vi "input to tag bus.vi"(9 "indices":T1, 10 "data cluster":T2, 11 "tag bus in":T3) -> (3 "tag bus out":T3)   [LabVIEW 2017, in "GPIC Core runtime.lvclass"]
uses:
  GPIC Core runtime.lvclass
  <vilib>/NI/Tag Bus/table/data table.ctl
  input user data.ctl
  configuration/input data indices.ctl
  <vilib>/NI/Tag Bus/table/data polymorphs/write one/write Boolean.vi
  <vilib>/NI/Tag Bus/table/data polymorphs/write one/write Single.vi
  <vilib>/NI/Tag Bus/table/data polymorphs/write one/write I16.vi
  <vilib>/NI/Tag Bus/table/data table.lvlib
  configuration/GPIC Core configuration.lvclass
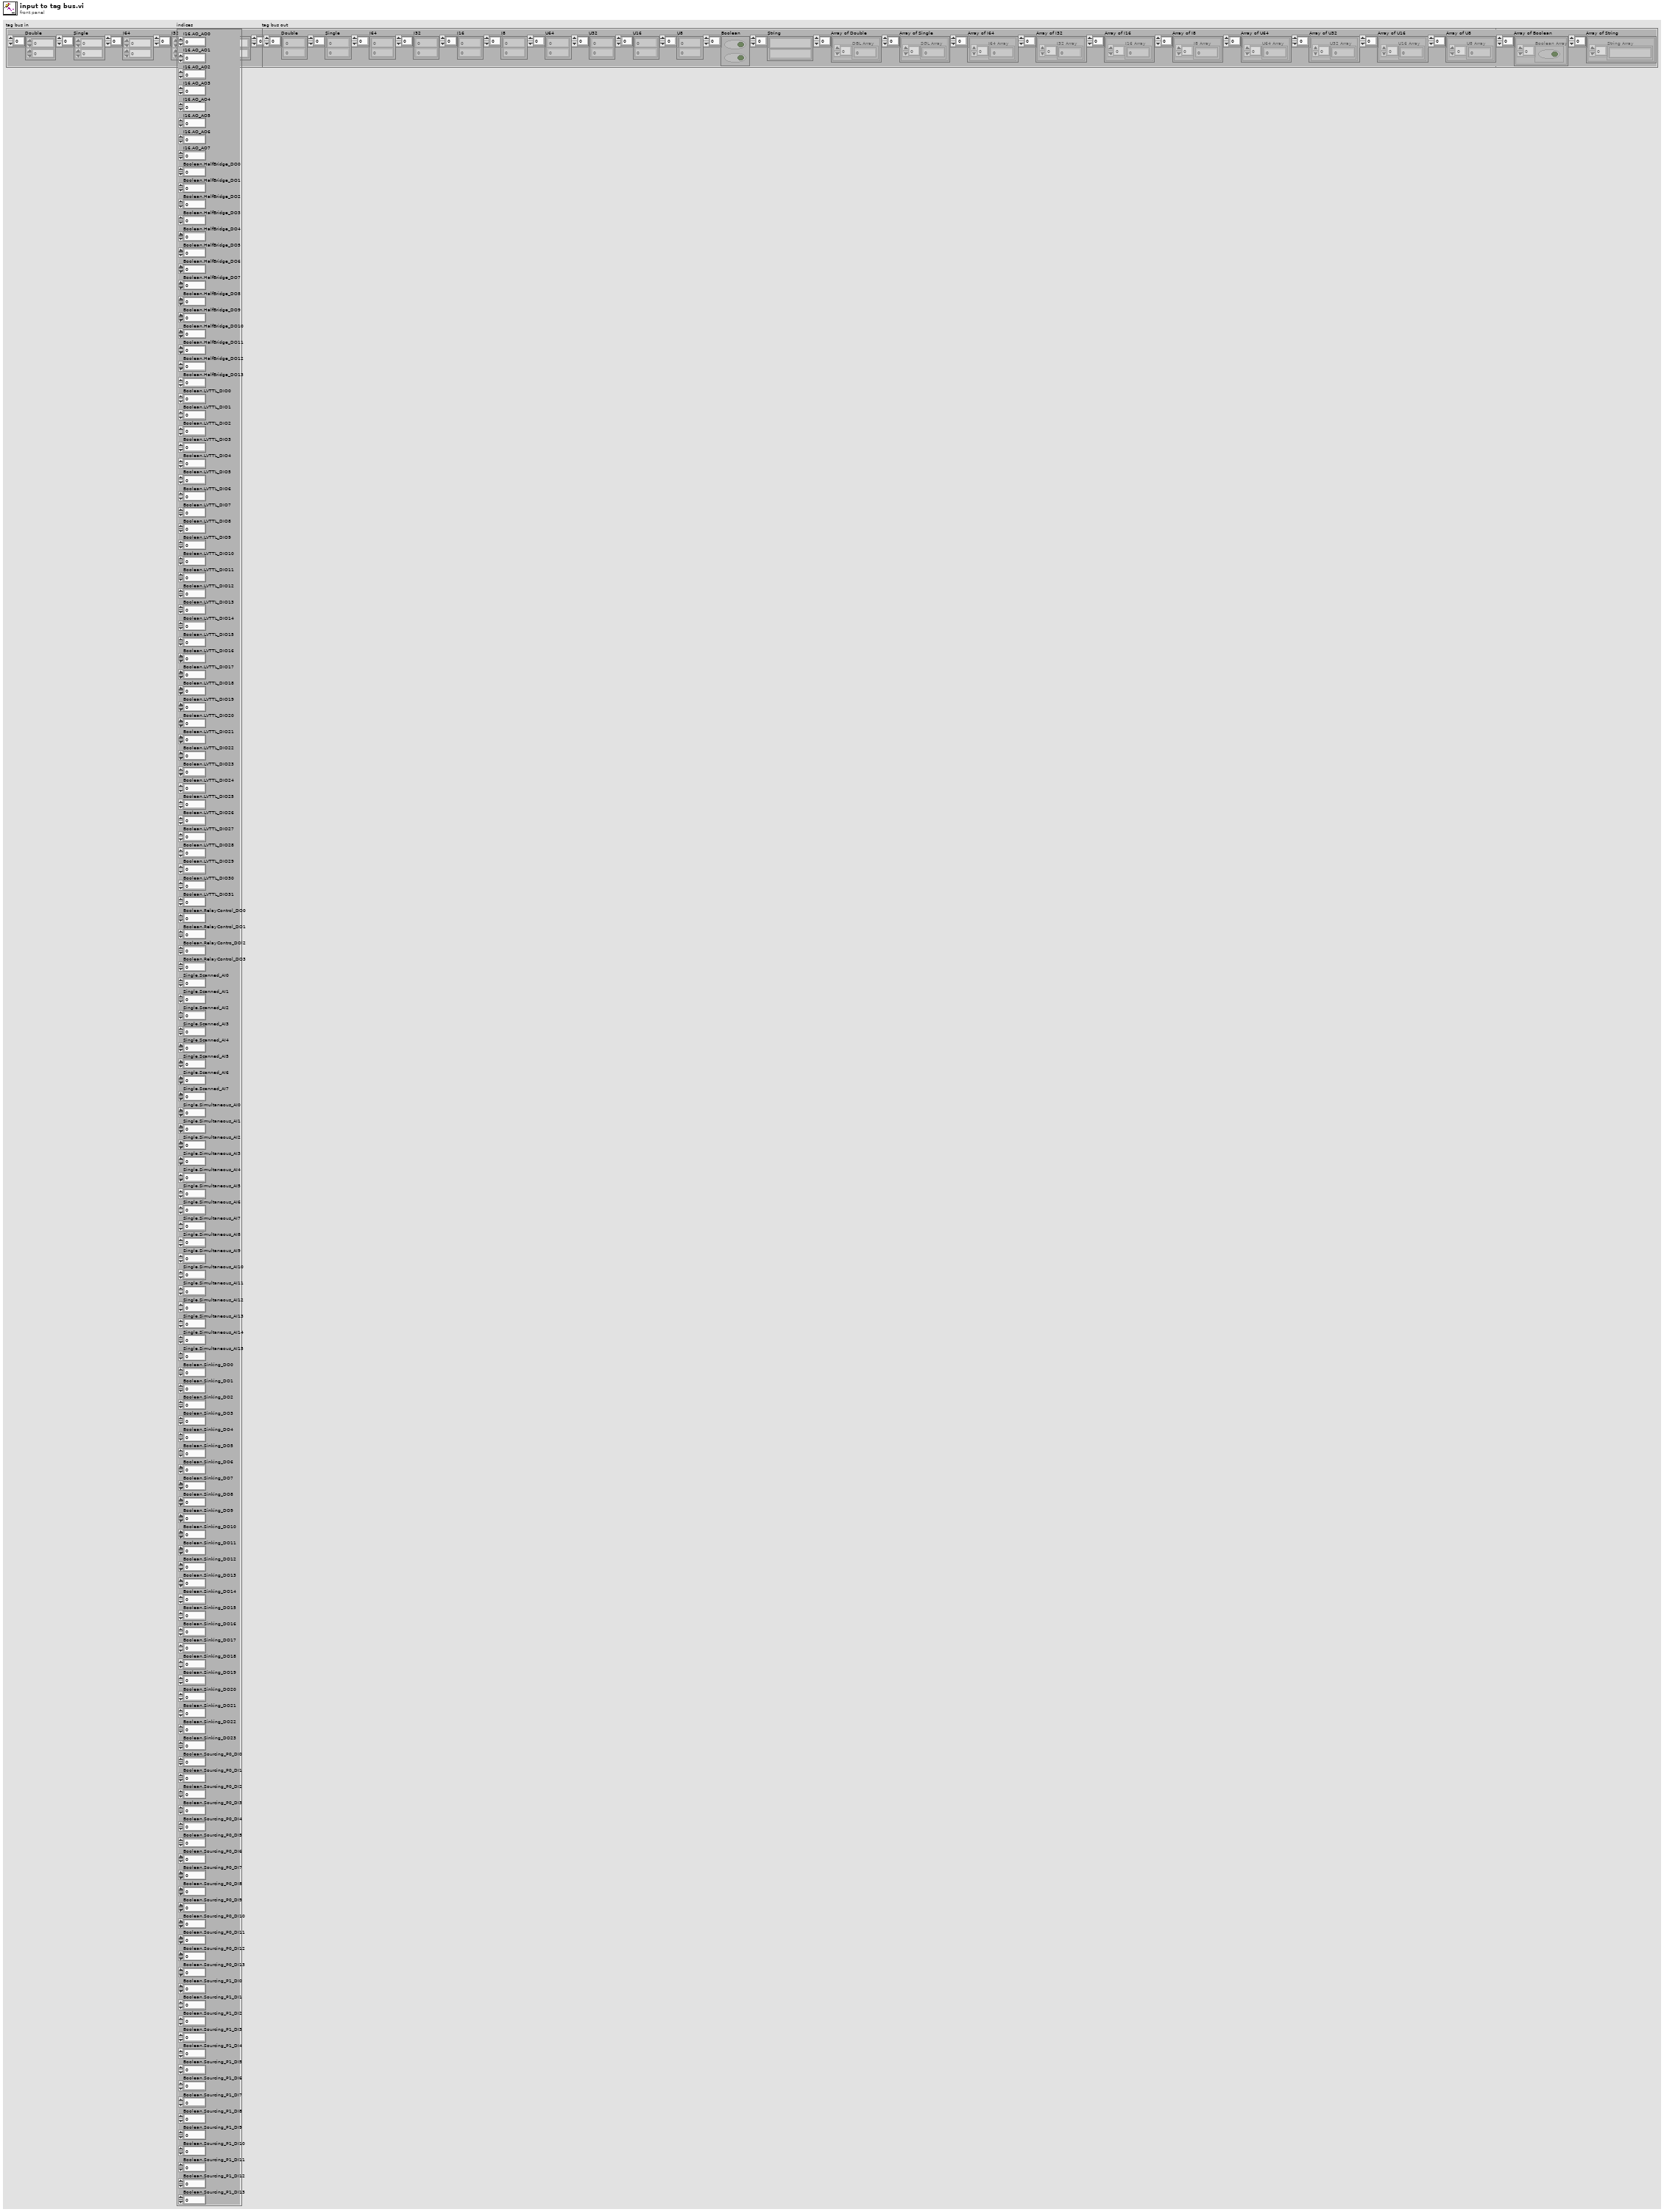
[diagram p1: front panel]
types:
  T1 = typedef "GPIC Core configuration.lvclass/input data indices.ctl" = cluster{"I16.AO_AO0":i32, "I16.AO_AO1":i32, "I16.AO_AO2":i32, "I16.AO_AO3":i32, "I16.AO_AO4":i32, "I16.AO_AO5":i32, "I16.AO_AO6":i32, "I16.AO_AO7":i32, "Boolean.HalfBridge_DO0":i32, "Boolean.HalfBridge_DO1":i32, "Boolean.HalfBridge_DO2":i32, "Boolean.HalfBridge_DO3":i32, "Boolean.HalfBridge_DO4":i32, "Boolean.HalfBridge_DO5":i32, "Boolean.HalfBridge_DO6":i32, "Boolean.HalfBridge_DO7":i32, "Boolean.HalfBridge_DO8":i32, "Boolean.HalfBridge_DO9":i32, "Boolean.HalfBridge_DO10":i32, "Boolean.HalfBridge_DO11":i32, "Boolean.HalfBridge_DO12":i32, "Boolean.HalfBridge_DO13":i32, "Boolean.LVTTL_DIO0":i32, "Boolean.LVTTL_DIO1":i32, "Boolean.LVTTL_DIO2":i32, "Boolean.LVTTL_DIO3":i32, "Boolean.LVTTL_DIO4":i32, "Boolean.LVTTL_DIO5":i32, "Boolean.LVTTL_DIO6":i32, "Boolean.LVTTL_DIO7":i32, "Boolean.LVTTL_DIO8":i32, "Boolean.LVTTL_DIO9":i32, "Boolean.LVTTL_DIO10":i32, "Boolean.LVTTL_DIO11":i32, "Boolean.LVTTL_DIO12":i32, "Boolean.LVTTL_DIO13":i32, "Boolean.LVTTL_DIO14":i32, "Boolean.LVTTL_DIO15":i32, "Boolean.LVTTL_DIO16":i32, "Boolean.LVTTL_DIO17":i32, "Boolean.LVTTL_DIO18":i32, "Boolean.LVTTL_DIO19":i32, "Boolean.LVTTL_DIO20":i32, "Boolean.LVTTL_DIO21":i32, "Boolean.LVTTL_DIO22":i32, "Boolean.LVTTL_DIO23":i32, "Boolean.LVTTL_DIO24":i32, "Boolean.LVTTL_DIO25":i32, "Boolean.LVTTL_DIO26":i32, "Boolean.LVTTL_DIO27":i32, "Boolean.LVTTL_DIO28":i32, "Boolean.LVTTL_DIO29":i32, "Boolean.LVTTL_DIO30":i32, "Boolean.LVTTL_DIO31":i32, "Boolean.RelayControl_DO0":i32, "Boolean.RelayControl_DO1":i32, "Boolean.RelayContro_DOl2":i32, "Boolean.RelayControl_DO3":i32, "Single.Scanned_AI0":i32, "Single.Scanned_AI1":i32, "Single.Scanned_AI2":i32, "Single.Scanned_AI3":i32, "Single.Scanned_AI4":i32, "Single.Scanned_AI5":i32, "Single.Scanned_AI6":i32, "Single.Scanned_AI7":i32, "Single.Simultaneous_AI0":i32, "Single.Simultaneous_AI1":i32, "Single.Simultaneous_AI2":i32, "Single.Simultaneous_AI3":i32, "Single.Simultaneous_AI4":i32, "Single.Simultaneous_AI5":i32, "Single.Simultaneous_AI6":i32, "Single.Simultaneous_AI7":i32, "Single.Simultaneous_AI8":i32, "Single.Simultaneous_AI9":i32, "Single.Simultaneous_AI10":i32, "Single.Simultaneous_AI11":i32, "Single.Simultaneous_AI12":i32, "Single.Simultaneous_AI13":i32, "Single.Simultaneous_AI14":i32, "Single.Simultaneous_AI15":i32, "Boolean.Sinking_DO0":i32, "Boolean.Sinking_DO1":i32, "Boolean.Sinking_DO2":i32, "Boolean.Sinking_DO3":i32, "Boolean.Sinking_DO4":i32, "Boolean.Sinking_DO5":i32, "Boolean.Sinking_DO6":i32, "Boolean.Sinking_DO7":i32, "Boolean.Sinking_DO8":i32, "Boolean.Sinking_DO9":i32, "Boolean.Sinking_DO10":i32, "Boolean.Sinking_DO11":i32, "Boolean.Sinking_DO12":i32, "Boolean.Sinking_DO13":i32, "Boolean.Sinking_DO14":i32, "Boolean.Sinking_DO15":i32, "Boolean.Sinking_DO16":i32, "Boolean.Sinking_DO17":i32, "Boolean.Sinking_DO18":i32, "Boolean.Sinking_DO19":i32, "Boolean.Sinking_DO20":i32, "Boolean.Sinking_DO21":i32, "Boolean.Sinking_DO22":i32, "Boolean.Sinking_DO23":i32, "Boolean.Sourcing_P0_DI0":i32, "Boolean.Sourcing_P0_DI1":i32, "Boolean.Sourcing_P0_DI2":i32, "Boolean.Sourcing_P0_DI3":i32, "Boolean.Sourcing_P0_DI4":i32, "Boolean.Sourcing_P0_DI5":i32, "Boolean.Sourcing_P0_DI6":i32, "Boolean.Sourcing_P0_DI7":i32, "Boolean.Sourcing_P0_DI8":i32, "Boolean.Sourcing_P0_DI9":i32, "Boolean.Sourcing_P0_DI10":i32, "Boolean.Sourcing_P0_DI11":i32, "Boolean.Sourcing_P0_DI12":i32, "Boolean.Sourcing_P0_DI13":i32, "Boolean.Sourcing_P1_DI0":i32, "Boolean.Sourcing_P1_DI1":i32, "Boolean.Sourcing_P1_DI2":i32, "Boolean.Sourcing_P1_DI3":i32, "Boolean.Sourcing_P1_DI4":i32, "Boolean.Sourcing_P1_DI5":i32, "Boolean.Sourcing_P1_DI6":i32, "Boolean.Sourcing_P1_DI7":i32, "Boolean.Sourcing_P1_DI8":i32, "Boolean.Sourcing_P1_DI9":i32, "Boolean.Sourcing_P1_DI10":i32, "Boolean.Sourcing_P1_DI11":i32, "Boolean.Sourcing_P1_DI12":i32, "Boolean.Sourcing_P1_DI13":i32}
  T2 = typedef "GPIC Core runtime.lvclass/input user data.ctl" = cluster{"AO_AO0":i16, "AO_AO1":i16, "AO_AO2":i16, "AO_AO3":i16, "AO_AO4":i16, "AO_AO5":i16, "AO_AO6":i16, "AO_AO7":i16, "HalfBridge_DO0":bool, "HalfBridge_DO1":bool, "HalfBridge_DO2":bool, "HalfBridge_DO3":bool, "HalfBridge_DO4":bool, "HalfBridge_DO5":bool, "HalfBridge_DO6":bool, "HalfBridge_DO7":bool, "HalfBridge_DO8":bool, "HalfBridge_DO9":bool, "HalfBridge_DO10":bool, "HalfBridge_DO11":bool, "HalfBridge_DO12":bool, "HalfBridge_DO13":bool, "LVTTL_DIO0":bool, "LVTTL_DIO1":bool, "LVTTL_DIO2":bool, "LVTTL_DIO3":bool, "LVTTL_DIO4":bool, "LVTTL_DIO5":bool, "LVTTL_DIO6":bool, "LVTTL_DIO7":bool, "LVTTL_DIO8":bool, "LVTTL_DIO9":bool, "LVTTL_DIO10":bool, "LVTTL_DIO11":bool, "LVTTL_DIO12":bool, "LVTTL_DIO13":bool, "LVTTL_DIO14":bool, "LVTTL_DIO15":bool, "LVTTL_DIO16":bool, "LVTTL_DIO17":bool, "LVTTL_DIO18":bool, "LVTTL_DIO19":bool, "LVTTL_DIO20":bool, "LVTTL_DIO21":bool, "LVTTL_DIO22":bool, "LVTTL_DIO23":bool, "LVTTL_DIO24":bool, "LVTTL_DIO25":bool, "LVTTL_DIO26":bool, "LVTTL_DIO27":bool, "LVTTL_DIO28":bool, "LVTTL_DIO29":bool, "LVTTL_DIO30":bool, "LVTTL_DIO31":bool, "RelayControl_DO0":bool, "RelayControl_DO1":bool, "RelayContro_DOl2":bool, "RelayControl_DO3":bool, "Scanned_AI0":sgl, "Scanned_AI1":sgl, "Scanned_AI2":sgl, "Scanned_AI3":sgl, "Scanned_AI4":sgl, "Scanned_AI5":sgl, "Scanned_AI6":sgl, "Scanned_AI7":sgl, "Simultaneous_AI0":sgl, "Simultaneous_AI1":sgl, "Simultaneous_AI2":sgl, "Simultaneous_AI3":sgl, "Simultaneous_AI4":sgl, "Simultaneous_AI5":sgl, "Simultaneous_AI6":sgl, "Simultaneous_AI7":sgl, "Simultaneous_AI8":sgl, "Simultaneous_AI9":sgl, "Simultaneous_AI10":sgl, "Simultaneous_AI11":sgl, "Simultaneous_AI12":sgl, "Simultaneous_AI13":sgl, "Simultaneous_AI14":sgl, "Simultaneous_AI15":sgl, "Sinking_DO0":bool, "Sinking_DO1":bool, "Sinking_DO2":bool, "Sinking_DO3":bool, "Sinking_DO4":bool, "Sinking_DO5":bool, "Sinking_DO6":bool, "Sinking_DO7":bool, "Sinking_DO8":bool, "Sinking_DO9":bool, "Sinking_DO10":bool, "Sinking_DO11":bool, "Sinking_DO12":bool, "Sinking_DO13":bool, "Sinking_DO14":bool, "Sinking_DO15":bool, "Sinking_DO16":bool, "Sinking_DO17":bool, "Sinking_DO18":bool, "Sinking_DO19":bool, "Sinking_DO20":bool, "Sinking_DO21":bool, "Sinking_DO22":bool, "Sinking_DO23":bool, "Sourcing_P0_DI0":bool, "Sourcing_P0_DI1":bool, "Sourcing_P0_DI2":bool, "Sourcing_P0_DI3":bool, "Sourcing_P0_DI4":bool, "Sourcing_P0_DI5":bool, "Sourcing_P0_DI6":bool, "Sourcing_P0_DI7":bool, "Sourcing_P0_DI8":bool, "Sourcing_P0_DI9":bool, "Sourcing_P0_DI10":bool, "Sourcing_P0_DI11":bool, "Sourcing_P0_DI12":bool, "Sourcing_P0_DI13":bool, "Sourcing_P1_DI0":bool, "Sourcing_P1_DI1":bool, "Sourcing_P1_DI2":bool, "Sourcing_P1_DI3":bool, "Sourcing_P1_DI4":bool, "Sourcing_P1_DI5":bool, "Sourcing_P1_DI6":bool, "Sourcing_P1_DI7":bool, "Sourcing_P1_DI8":bool, "Sourcing_P1_DI9":bool, "Sourcing_P1_DI10":bool, "Sourcing_P1_DI11":bool, "Sourcing_P1_DI12":bool, "Sourcing_P1_DI13":bool}
  T3 = typedef "tag bus.lvlib/data table.lvlib/data table.ctl" = cluster{"Double":dbl[], "Single":sgl[], "I64":i64[], "I32":i32[], "I16":i16[], "I8":i8[], "U64":u64[], "U32":u32[], "U16":u16[], "U8":u8[], "Boolean":bool[], "String":string[], "Array of Double":cluster{"DBL Array":dbl[]}[], "Array of Single":cluster{"SGL Array":sgl[]}[], "Array of I64":cluster{"I64 Array":i64[]}[], "Array of I32":cluster{"I32 Array":i32[]}[], "Array of I16":cluster{"I16 Array":i16[]}[], "Array of I8":cluster{"I8 Array":i8[]}[], "Array of U64":cluster{"U64 Array":u64[]}[], "Array of U32":cluster{"U32 Array":u32[]}[], "Array of U16":cluster{"U16 Array":u16[]}[], "Array of U8":cluster{"U8 Array":u8[]}[], "Array of Boolean":cluster{"Boolean Array":bool[]}[], "Array of String":cluster{"String Array":string[]}[]}
diagram:
  n1 = Unbundle By Name("indices") -> ("I16.AO_AO0"=w4:i32, "I16.AO_AO1"=w7:i32, "I16.AO_AO2"=w10:i32, "I16.AO_AO3"=w13:i32, "I16.AO_AO4"=w16:i32, "I16.AO_AO5"=w19:i32, "I16.AO_AO6"=w22:i32, "I16.AO_AO7"=w25:i32, "Boolean.HalfBridge_DO0"=w28:i32, "Boolean.HalfBridge_DO1"=w31:i32, "Boolean.HalfBridge_DO2"=w34:i32, "Boolean.HalfBridge_DO3"=w37:i32, "Boolean.HalfBridge_DO4"=w40:i32, "Boolean.HalfBridge_DO5"=w43:i32, "Boolean.HalfBridge_DO6"=w46:i32, "Boolean.HalfBridge_DO7"=w49:i32, "Boolean.HalfBridge_DO8"=w52:i32, "Boolean.HalfBridge_DO9"=w55:i32, "Boolean.HalfBridge_DO10"=w58:i32, "Boolean.HalfBridge_DO11"=w61:i32, "Boolean.HalfBridge_DO12"=w64:i32, "Boolean.HalfBridge_DO13"=w67:i32, "Boolean.LVTTL_DIO0"=w70:i32, "Boolean.LVTTL_DIO1"=w73:i32, "Boolean.LVTTL_DIO2"=w76:i32, "Boolean.LVTTL_DIO3"=w79:i32, "Boolean.LVTTL_DIO4"=w82:i32, "Boolean.LVTTL_DIO5"=w85:i32, "Boolean.LVTTL_DIO6"=w88:i32, "Boolean.LVTTL_DIO7"=w91:i32, "Boolean.LVTTL_DIO8"=w94:i32, "Boolean.LVTTL_DIO9"=w97:i32, "Boolean.LVTTL_DIO10"=w100:i32, "Boolean.LVTTL_DIO11"=w103:i32, "Boolean.LVTTL_DIO12"=w106:i32, "Boolean.LVTTL_DIO13"=w109:i32, "Boolean.LVTTL_DIO14"=w112:i32, "Boolean.LVTTL_DIO15"=w115:i32, "Boolean.LVTTL_DIO16"=w118:i32, "Boolean.LVTTL_DIO17"=w121:i32, "Boolean.LVTTL_DIO18"=w124:i32, "Boolean.LVTTL_DIO19"=w127:i32, "Boolean.LVTTL_DIO20"=w130:i32, "Boolean.LVTTL_DIO21"=w133:i32, "Boolean.LVTTL_DIO22"=w136:i32, "Boolean.LVTTL_DIO23"=w139:i32, "Boolean.LVTTL_DIO24"=w142:i32, "Boolean.LVTTL_DIO25"=w145:i32, "Boolean.LVTTL_DIO26"=w148:i32, "Boolean.LVTTL_DIO27"=w151:i32, "Boolean.LVTTL_DIO28"=w154:i32, "Boolean.LVTTL_DIO29"=w157:i32, "Boolean.LVTTL_DIO30"=w160:i32, "Boolean.LVTTL_DIO31"=w163:i32, "Boolean.RelayControl_DO0"=w166:i32, "Boolean.RelayControl_DO1"=w169:i32, "Boolean.RelayContro_DOl2"=w172:i32, "Boolean.RelayControl_DO3"=w175:i32, "Single.Scanned_AI0"=w178:i32, "Single.Scanned_AI1"=w181:i32, "Single.Scanned_AI2"=w184:i32, "Single.Scanned_AI3"=w187:i32, "Single.Scanned_AI4"=w190:i32, "Single.Scanned_AI5"=w193:i32, "Single.Scanned_AI6"=w196:i32, "Single.Scanned_AI7"=w199:i32, "Single.Simultaneous_AI0"=w202:i32, "Single.Simultaneous_AI1"=w205:i32, "Single.Simultaneous_AI2"=w208:i32, "Single.Simultaneous_AI3"=w211:i32, "Single.Simultaneous_AI4"=w214:i32, "Single.Simultaneous_AI5"=w217:i32, "Single.Simultaneous_AI6"=w220:i32, "Single.Simultaneous_AI7"=w223:i32, "Single.Simultaneous_AI8"=w226:i32, "Single.Simultaneous_AI9"=w229:i32, "Single.Simultaneous_AI10"=w232:i32, "Single.Simultaneous_AI11"=w235:i32, "Single.Simultaneous_AI12"=w238:i32, "Single.Simultaneous_AI13"=w241:i32, "Single.Simultaneous_AI14"=w244:i32, "Single.Simultaneous_AI15"=w247:i32, "Boolean.Sinking_DO0"=w250:i32, "Boolean.Sinking_DO1"=w253:i32, "Boolean.Sinking_DO2"=w256:i32, "Boolean.Sinking_DO3"=w259:i32, "Boolean.Sinking_DO4"=w262:i32, "Boolean.Sinking_DO5"=w265:i32, "Boolean.Sinking_DO6"=w268:i32, "Boolean.Sinking_DO7"=w271:i32, "Boolean.Sinking_DO8"=w274:i32, "Boolean.Sinking_DO9"=w277:i32, "Boolean.Sinking_DO10"=w280:i32, "Boolean.Sinking_DO11"=w283:i32, "Boolean.Sinking_DO12"=w286:i32, "Boolean.Sinking_DO13"=w289:i32, "Boolean.Sinking_DO14"=w292:i32, "Boolean.Sinking_DO15"=w295:i32, "Boolean.Sinking_DO16"=w298:i32, "Boolean.Sinking_DO17"=w301:i32, "Boolean.Sinking_DO18"=w304:i32, "Boolean.Sinking_DO19"=w307:i32, "Boolean.Sinking_DO20"=w310:i32, "Boolean.Sinking_DO21"=w313:i32, "Boolean.Sinking_DO22"=w316:i32, "Boolean.Sinking_DO23"=w319:i32, "Boolean.Sourcing_P0_DI0"=w322:i32, "Boolean.Sourcing_P0_DI1"=w325:i32, "Boolean.Sourcing_P0_DI2"=w328:i32, "Boolean.Sourcing_P0_DI3"=w331:i32, "Boolean.Sourcing_P0_DI4"=w334:i32, "Boolean.Sourcing_P0_DI5"=w337:i32, "Boolean.Sourcing_P0_DI6"=w340:i32, "Boolean.Sourcing_P0_DI7"=w343:i32, "Boolean.Sourcing_P0_DI8"=w346:i32, "Boolean.Sourcing_P0_DI9"=w349:i32, "Boolean.Sourcing_P0_DI10"=w352:i32, "Boolean.Sourcing_P0_DI11"=w355:i32, "Boolean.Sourcing_P0_DI12"=w358:i32, "Boolean.Sourcing_P0_DI13"=w361:i32, "Boolean.Sourcing_P1_DI0"=w364:i32, "Boolean.Sourcing_P1_DI1"=w367:i32, "Boolean.Sourcing_P1_DI2"=w370:i32, "Boolean.Sourcing_P1_DI3"=w373:i32, "Boolean.Sourcing_P1_DI4"=w376:i32, "Boolean.Sourcing_P1_DI5"=w379:i32, "Boolean.Sourcing_P1_DI6"=w382:i32, "Boolean.Sourcing_P1_DI7"=w385:i32, "Boolean.Sourcing_P1_DI8"=w388:i32, "Boolean.Sourcing_P1_DI9"=w391:i32, "Boolean.Sourcing_P1_DI10"=w394:i32, "Boolean.Sourcing_P1_DI11"=w397:i32, "Boolean.Sourcing_P1_DI12"=w400:i32, "Boolean.Sourcing_P1_DI13"=w403:i32)
  n2 = Unbundle By Name("data cluster") -> ("AO_AO0"=w3:i16, "AO_AO1"=w6:i16, "AO_AO2"=w9:i16, "AO_AO3"=w12:i16, "AO_AO4"=w15:i16, "AO_AO5"=w18:i16, "AO_AO6"=w21:i16, "AO_AO7"=w24:i16, "HalfBridge_DO0"=w27:bool, "HalfBridge_DO1"=w30:bool, "HalfBridge_DO2"=w33:bool, "HalfBridge_DO3"=w36:bool, "HalfBridge_DO4"=w39:bool, "HalfBridge_DO5"=w42:bool, "HalfBridge_DO6"=w45:bool, "HalfBridge_DO7"=w48:bool, "HalfBridge_DO8"=w51:bool, "HalfBridge_DO9"=w54:bool, "HalfBridge_DO10"=w57:bool, "HalfBridge_DO11"=w60:bool, "HalfBridge_DO12"=w63:bool, "HalfBridge_DO13"=w66:bool, "LVTTL_DIO0"=w69:bool, "LVTTL_DIO1"=w72:bool, "LVTTL_DIO2"=w75:bool, "LVTTL_DIO3"=w78:bool, "LVTTL_DIO4"=w81:bool, "LVTTL_DIO5"=w84:bool, "LVTTL_DIO6"=w87:bool, "LVTTL_DIO7"=w90:bool, "LVTTL_DIO8"=w93:bool, "LVTTL_DIO9"=w96:bool, "LVTTL_DIO10"=w99:bool, "LVTTL_DIO11"=w102:bool, "LVTTL_DIO12"=w105:bool, "LVTTL_DIO13"=w108:bool, "LVTTL_DIO14"=w111:bool, "LVTTL_DIO15"=w114:bool, "LVTTL_DIO16"=w117:bool, "LVTTL_DIO17"=w120:bool, "LVTTL_DIO18"=w123:bool, "LVTTL_DIO19"=w126:bool, "LVTTL_DIO20"=w129:bool, "LVTTL_DIO21"=w132:bool, "LVTTL_DIO22"=w135:bool, "LVTTL_DIO23"=w138:bool, "LVTTL_DIO24"=w141:bool, "LVTTL_DIO25"=w144:bool, "LVTTL_DIO26"=w147:bool, "LVTTL_DIO27"=w150:bool, "LVTTL_DIO28"=w153:bool, "LVTTL_DIO29"=w156:bool, "LVTTL_DIO30"=w159:bool, "LVTTL_DIO31"=w162:bool, "RelayControl_DO0"=w165:bool, "RelayControl_DO1"=w168:bool, "RelayContro_DOl2"=w171:bool, "RelayControl_DO3"=w174:bool, "Scanned_AI0"=w177:sgl, "Scanned_AI1"=w180:sgl, "Scanned_AI2"=w183:sgl, "Scanned_AI3"=w186:sgl, "Scanned_AI4"=w189:sgl, "Scanned_AI5"=w192:sgl, "Scanned_AI6"=w195:sgl, "Scanned_AI7"=w198:sgl, "Simultaneous_AI0"=w201:sgl, "Simultaneous_AI1"=w204:sgl, "Simultaneous_AI2"=w207:sgl, "Simultaneous_AI3"=w210:sgl, "Simultaneous_AI4"=w213:sgl, "Simultaneous_AI5"=w216:sgl, "Simultaneous_AI6"=w219:sgl, "Simultaneous_AI7"=w222:sgl, "Simultaneous_AI8"=w225:sgl, "Simultaneous_AI9"=w228:sgl, "Simultaneous_AI10"=w231:sgl, "Simultaneous_AI11"=w234:sgl, "Simultaneous_AI12"=w237:sgl, "Simultaneous_AI13"=w240:sgl, "Simultaneous_AI14"=w243:sgl, "Simultaneous_AI15"=w246:sgl, "Sinking_DO0"=w249:bool, "Sinking_DO1"=w252:bool, "Sinking_DO2"=w255:bool, "Sinking_DO3"=w258:bool, "Sinking_DO4"=w261:bool, "Sinking_DO5"=w264:bool, "Sinking_DO6"=w267:bool, "Sinking_DO7"=w270:bool, "Sinking_DO8"=w273:bool, "Sinking_DO9"=w276:bool, "Sinking_DO10"=w279:bool, "Sinking_DO11"=w282:bool, "Sinking_DO12"=w285:bool, "Sinking_DO13"=w288:bool, "Sinking_DO14"=w291:bool, "Sinking_DO15"=w294:bool, "Sinking_DO16"=w297:bool, "Sinking_DO17"=w300:bool, "Sinking_DO18"=w303:bool, "Sinking_DO19"=w306:bool, "Sinking_DO20"=w309:bool, "Sinking_DO21"=w312:bool, "Sinking_DO22"=w315:bool, "Sinking_DO23"=w318:bool, "Sourcing_P0_DI0"=w321:bool, "Sourcing_P0_DI1"=w324:bool, "Sourcing_P0_DI2"=w327:bool, "Sourcing_P0_DI3"=w330:bool, "Sourcing_P0_DI4"=w333:bool, "Sourcing_P0_DI5"=w336:bool, "Sourcing_P0_DI6"=w339:bool, "Sourcing_P0_DI7"=w342:bool, "Sourcing_P0_DI8"=w345:bool, "Sourcing_P0_DI9"=w348:bool, "Sourcing_P0_DI10"=w351:bool, "Sourcing_P0_DI11"=w354:bool, "Sourcing_P0_DI12"=w357:bool, "Sourcing_P0_DI13"=w360:bool, "Sourcing_P1_DI0"=w363:bool, "Sourcing_P1_DI1"=w366:bool, "Sourcing_P1_DI2"=w369:bool, "Sourcing_P1_DI3"=w372:bool, "Sourcing_P1_DI4"=w375:bool, "Sourcing_P1_DI5"=w378:bool, "Sourcing_P1_DI6"=w381:bool, "Sourcing_P1_DI7"=w384:bool, "Sourcing_P1_DI8"=w387:bool, "Sourcing_P1_DI9"=w390:bool, "Sourcing_P1_DI10"=w393:bool, "Sourcing_P1_DI11"=w396:bool, "Sourcing_P1_DI12"=w399:bool, "Sourcing_P1_DI13"=w402:bool)
  n3 = call-poly <vilib>:"write data element.vi"("value"=w402, "index"=w403, "data table in"="tag bus in") -> ("data table out"=w398:T3)  [unwired: 8 in]
  n4 = call-poly <vilib>:"write data element.vi"("value"=w399, "index"=w400, "data table in"=w398) -> ("data table out"=w395:T3)  [unwired: 8 in]
  n5 = call-poly <vilib>:"write data element.vi"("value"=w396, "index"=w397, "data table in"=w395) -> ("data table out"=w392:T3)  [unwired: 8 in]
  n6 = call-poly <vilib>:"write data element.vi"("value"=w393, "index"=w394, "data table in"=w392) -> ("data table out"=w389:T3)  [unwired: 8 in]
  n7 = call-poly <vilib>:"write data element.vi"("value"=w390, "index"=w391, "data table in"=w389) -> ("data table out"=w386:T3)  [unwired: 8 in]
  n8 = call-poly <vilib>:"write data element.vi"("value"=w387, "index"=w388, "data table in"=w386) -> ("data table out"=w383:T3)  [unwired: 8 in]
  n9 = call-poly <vilib>:"write data element.vi"("value"=w384, "index"=w385, "data table in"=w383) -> ("data table out"=w380:T3)  [unwired: 8 in]
  n10 = call-poly <vilib>:"write data element.vi"("value"=w381, "index"=w382, "data table in"=w380) -> ("data table out"=w377:T3)  [unwired: 8 in]
  n11 = call-poly <vilib>:"write data element.vi"("value"=w378, "index"=w379, "data table in"=w377) -> ("data table out"=w374:T3)  [unwired: 8 in]
  n12 = call-poly <vilib>:"write data element.vi"("value"=w375, "index"=w376, "data table in"=w374) -> ("data table out"=w371:T3)  [unwired: 8 in]
  n13 = call-poly <vilib>:"write data element.vi"("value"=w372, "index"=w373, "data table in"=w371) -> ("data table out"=w368:T3)  [unwired: 8 in]
  n14 = call-poly <vilib>:"write data element.vi"("value"=w369, "index"=w370, "data table in"=w368) -> ("data table out"=w365:T3)  [unwired: 8 in]
  n15 = call-poly <vilib>:"write data element.vi"("value"=w366, "index"=w367, "data table in"=w365) -> ("data table out"=w362:T3)  [unwired: 8 in]
  n16 = call-poly <vilib>:"write data element.vi"("value"=w363, "index"=w364, "data table in"=w362) -> ("data table out"=w359:T3)  [unwired: 8 in]
  n17 = call-poly <vilib>:"write data element.vi"("value"=w360, "index"=w361, "data table in"=w359) -> ("data table out"=w356:T3)  [unwired: 8 in]
  n18 = call-poly <vilib>:"write data element.vi"("value"=w357, "index"=w358, "data table in"=w356) -> ("data table out"=w353:T3)  [unwired: 8 in]
  n19 = call-poly <vilib>:"write data element.vi"("value"=w354, "index"=w355, "data table in"=w353) -> ("data table out"=w350:T3)  [unwired: 8 in]
  n20 = call-poly <vilib>:"write data element.vi"("value"=w351, "index"=w352, "data table in"=w350) -> ("data table out"=w347:T3)  [unwired: 8 in]
  n21 = call-poly <vilib>:"write data element.vi"("value"=w348, "index"=w349, "data table in"=w347) -> ("data table out"=w344:T3)  [unwired: 8 in]
  n22 = call-poly <vilib>:"write data element.vi"("value"=w345, "index"=w346, "data table in"=w344) -> ("data table out"=w341:T3)  [unwired: 8 in]
  n23 = call-poly <vilib>:"write data element.vi"("value"=w342, "index"=w343, "data table in"=w341) -> ("data table out"=w338:T3)  [unwired: 8 in]
  n24 = call-poly <vilib>:"write data element.vi"("value"=w339, "index"=w340, "data table in"=w338) -> ("data table out"=w335:T3)  [unwired: 8 in]
  n25 = call-poly <vilib>:"write data element.vi"("value"=w336, "index"=w337, "data table in"=w335) -> ("data table out"=w332:T3)  [unwired: 8 in]
  n26 = call-poly <vilib>:"write data element.vi"("value"=w333, "index"=w334, "data table in"=w332) -> ("data table out"=w329:T3)  [unwired: 8 in]
  n27 = call-poly <vilib>:"write data element.vi"("value"=w330, "index"=w331, "data table in"=w329) -> ("data table out"=w326:T3)  [unwired: 8 in]
  n28 = call-poly <vilib>:"write data element.vi"("value"=w327, "index"=w328, "data table in"=w326) -> ("data table out"=w323:T3)  [unwired: 8 in]
  n29 = call-poly <vilib>:"write data element.vi"("value"=w324, "index"=w325, "data table in"=w323) -> ("data table out"=w320:T3)  [unwired: 8 in]
  n30 = call-poly <vilib>:"write data element.vi"("value"=w321, "index"=w322, "data table in"=w320) -> ("data table out"=w317:T3)  [unwired: 8 in]
  n31 = call-poly <vilib>:"write data element.vi"("value"=w318, "index"=w319, "data table in"=w317) -> ("data table out"=w314:T3)  [unwired: 8 in]
  n32 = call-poly <vilib>:"write data element.vi"("value"=w315, "index"=w316, "data table in"=w314) -> ("data table out"=w311:T3)  [unwired: 8 in]
  n33 = call-poly <vilib>:"write data element.vi"("value"=w312, "index"=w313, "data table in"=w311) -> ("data table out"=w308:T3)  [unwired: 8 in]
  n34 = call-poly <vilib>:"write data element.vi"("value"=w309, "index"=w310, "data table in"=w308) -> ("data table out"=w305:T3)  [unwired: 8 in]
  n35 = call-poly <vilib>:"write data element.vi"("value"=w306, "index"=w307, "data table in"=w305) -> ("data table out"=w302:T3)  [unwired: 8 in]
  n36 = call-poly <vilib>:"write data element.vi"("value"=w303, "index"=w304, "data table in"=w302) -> ("data table out"=w299:T3)  [unwired: 8 in]
  n37 = call-poly <vilib>:"write data element.vi"("value"=w300, "index"=w301, "data table in"=w299) -> ("data table out"=w296:T3)  [unwired: 8 in]
  n38 = call-poly <vilib>:"write data element.vi"("value"=w297, "index"=w298, "data table in"=w296) -> ("data table out"=w293:T3)  [unwired: 8 in]
  n39 = call-poly <vilib>:"write data element.vi"("value"=w294, "index"=w295, "data table in"=w293) -> ("data table out"=w290:T3)  [unwired: 8 in]
  n40 = call-poly <vilib>:"write data element.vi"("value"=w291, "index"=w292, "data table in"=w290) -> ("data table out"=w287:T3)  [unwired: 8 in]
  n41 = call-poly <vilib>:"write data element.vi"("value"=w288, "index"=w289, "data table in"=w287) -> ("data table out"=w284:T3)  [unwired: 8 in]
  n42 = call-poly <vilib>:"write data element.vi"("value"=w285, "index"=w286, "data table in"=w284) -> ("data table out"=w281:T3)  [unwired: 8 in]
  n43 = call-poly <vilib>:"write data element.vi"("value"=w282, "index"=w283, "data table in"=w281) -> ("data table out"=w278:T3)  [unwired: 8 in]
  n44 = call-poly <vilib>:"write data element.vi"("value"=w279, "index"=w280, "data table in"=w278) -> ("data table out"=w275:T3)  [unwired: 8 in]
  n45 = call-poly <vilib>:"write data element.vi"("value"=w276, "index"=w277, "data table in"=w275) -> ("data table out"=w272:T3)  [unwired: 8 in]
  n46 = call-poly <vilib>:"write data element.vi"("value"=w273, "index"=w274, "data table in"=w272) -> ("data table out"=w269:T3)  [unwired: 8 in]
  n47 = call-poly <vilib>:"write data element.vi"("value"=w270, "index"=w271, "data table in"=w269) -> ("data table out"=w266:T3)  [unwired: 8 in]
  n48 = call-poly <vilib>:"write data element.vi"("value"=w267, "index"=w268, "data table in"=w266) -> ("data table out"=w263:T3)  [unwired: 8 in]
  n49 = call-poly <vilib>:"write data element.vi"("value"=w264, "index"=w265, "data table in"=w263) -> ("data table out"=w260:T3)  [unwired: 8 in]
  n50 = call-poly <vilib>:"write data element.vi"("value"=w261, "index"=w262, "data table in"=w260) -> ("data table out"=w257:T3)  [unwired: 8 in]
  n51 = call-poly <vilib>:"write data element.vi"("value"=w258, "index"=w259, "data table in"=w257) -> ("data table out"=w254:T3)  [unwired: 8 in]
  n52 = call-poly <vilib>:"write data element.vi"("value"=w255, "index"=w256, "data table in"=w254) -> ("data table out"=w251:T3)  [unwired: 8 in]
  n53 = call-poly <vilib>:"write data element.vi"("value"=w252, "index"=w253, "data table in"=w251) -> ("data table out"=w248:T3)  [unwired: 8 in]
  n54 = call-poly <vilib>:"write data element.vi"("value"=w249, "index"=w250, "data table in"=w248) -> ("data table out"=w245:T3)  [unwired: 8 in]
  n55 = call-poly <vilib>:"write data element.vi"("value"=w246, "index"=w247, "data table in"=w245) -> ("data table out"=w242:T3)  [unwired: 8 in]
  n56 = call-poly <vilib>:"write data element.vi"("value"=w243, "index"=w244, "data table in"=w242) -> ("data table out"=w239:T3)  [unwired: 8 in]
  n57 = call-poly <vilib>:"write data element.vi"("value"=w240, "index"=w241, "data table in"=w239) -> ("data table out"=w236:T3)  [unwired: 8 in]
  n58 = call-poly <vilib>:"write data element.vi"("value"=w237, "index"=w238, "data table in"=w236) -> ("data table out"=w233:T3)  [unwired: 8 in]
  n59 = call-poly <vilib>:"write data element.vi"("value"=w234, "index"=w235, "data table in"=w233) -> ("data table out"=w230:T3)  [unwired: 8 in]
  n60 = call-poly <vilib>:"write data element.vi"("value"=w231, "index"=w232, "data table in"=w230) -> ("data table out"=w227:T3)  [unwired: 8 in]
  n61 = call-poly <vilib>:"write data element.vi"("value"=w228, "index"=w229, "data table in"=w227) -> ("data table out"=w224:T3)  [unwired: 8 in]
  n62 = call-poly <vilib>:"write data element.vi"("value"=w225, "index"=w226, "data table in"=w224) -> ("data table out"=w221:T3)  [unwired: 8 in]
  n63 = call-poly <vilib>:"write data element.vi"("value"=w222, "index"=w223, "data table in"=w221) -> ("data table out"=w218:T3)  [unwired: 8 in]
  n64 = call-poly <vilib>:"write data element.vi"("value"=w219, "index"=w220, "data table in"=w218) -> ("data table out"=w215:T3)  [unwired: 8 in]
  n65 = call-poly <vilib>:"write data element.vi"("value"=w216, "index"=w217, "data table in"=w215) -> ("data table out"=w212:T3)  [unwired: 8 in]
  n66 = call-poly <vilib>:"write data element.vi"("value"=w213, "index"=w214, "data table in"=w212) -> ("data table out"=w209:T3)  [unwired: 8 in]
  n67 = call-poly <vilib>:"write data element.vi"("value"=w210, "index"=w211, "data table in"=w209) -> ("data table out"=w206:T3)  [unwired: 8 in]
  n68 = call-poly <vilib>:"write data element.vi"("value"=w207, "index"=w208, "data table in"=w206) -> ("data table out"=w203:T3)  [unwired: 8 in]
  n69 = call-poly <vilib>:"write data element.vi"("value"=w204, "index"=w205, "data table in"=w203) -> ("data table out"=w200:T3)  [unwired: 8 in]
  n70 = call-poly <vilib>:"write data element.vi"("value"=w201, "index"=w202, "data table in"=w200) -> ("data table out"=w197:T3)  [unwired: 8 in]
  n71 = call-poly <vilib>:"write data element.vi"("value"=w198, "index"=w199, "data table in"=w197) -> ("data table out"=w194:T3)  [unwired: 8 in]
  n72 = call-poly <vilib>:"write data element.vi"("value"=w195, "index"=w196, "data table in"=w194) -> ("data table out"=w191:T3)  [unwired: 8 in]
  n73 = call-poly <vilib>:"write data element.vi"("value"=w192, "index"=w193, "data table in"=w191) -> ("data table out"=w188:T3)  [unwired: 8 in]
  n74 = call-poly <vilib>:"write data element.vi"("value"=w189, "index"=w190, "data table in"=w188) -> ("data table out"=w185:T3)  [unwired: 8 in]
  n75 = call-poly <vilib>:"write data element.vi"("value"=w186, "index"=w187, "data table in"=w185) -> ("data table out"=w182:T3)  [unwired: 8 in]
  n76 = call-poly <vilib>:"write data element.vi"("value"=w183, "index"=w184, "data table in"=w182) -> ("data table out"=w179:T3)  [unwired: 8 in]
  n77 = call-poly <vilib>:"write data element.vi"("value"=w180, "index"=w181, "data table in"=w179) -> ("data table out"=w176:T3)  [unwired: 8 in]
  n78 = call-poly <vilib>:"write data element.vi"("value"=w177, "index"=w178, "data table in"=w176) -> ("data table out"=w173:T3)  [unwired: 8 in]
  n79 = call-poly <vilib>:"write data element.vi"("value"=w174, "index"=w175, "data table in"=w173) -> ("data table out"=w170:T3)  [unwired: 8 in]
  n80 = call-poly <vilib>:"write data element.vi"("value"=w171, "index"=w172, "data table in"=w170) -> ("data table out"=w167:T3)  [unwired: 8 in]
  n81 = call-poly <vilib>:"write data element.vi"("value"=w168, "index"=w169, "data table in"=w167) -> ("data table out"=w164:T3)  [unwired: 8 in]
  n82 = call-poly <vilib>:"write data element.vi"("value"=w165, "index"=w166, "data table in"=w164) -> ("data table out"=w161:T3)  [unwired: 8 in]
  n83 = call-poly <vilib>:"write data element.vi"("value"=w162, "index"=w163, "data table in"=w161) -> ("data table out"=w158:T3)  [unwired: 8 in]
  n84 = call-poly <vilib>:"write data element.vi"("value"=w159, "index"=w160, "data table in"=w158) -> ("data table out"=w155:T3)  [unwired: 8 in]
  n85 = call-poly <vilib>:"write data element.vi"("value"=w156, "index"=w157, "data table in"=w155) -> ("data table out"=w152:T3)  [unwired: 8 in]
  n86 = call-poly <vilib>:"write data element.vi"("value"=w153, "index"=w154, "data table in"=w152) -> ("data table out"=w149:T3)  [unwired: 8 in]
  n87 = call-poly <vilib>:"write data element.vi"("value"=w150, "index"=w151, "data table in"=w149) -> ("data table out"=w146:T3)  [unwired: 8 in]
  n88 = call-poly <vilib>:"write data element.vi"("value"=w147, "index"=w148, "data table in"=w146) -> ("data table out"=w143:T3)  [unwired: 8 in]
  n89 = call-poly <vilib>:"write data element.vi"("value"=w144, "index"=w145, "data table in"=w143) -> ("data table out"=w140:T3)  [unwired: 8 in]
  n90 = call-poly <vilib>:"write data element.vi"("value"=w141, "index"=w142, "data table in"=w140) -> ("data table out"=w137:T3)  [unwired: 8 in]
  n91 = call-poly <vilib>:"write data element.vi"("value"=w138, "index"=w139, "data table in"=w137) -> ("data table out"=w134:T3)  [unwired: 8 in]
  n92 = call-poly <vilib>:"write data element.vi"("value"=w135, "index"=w136, "data table in"=w134) -> ("data table out"=w131:T3)  [unwired: 8 in]
  n93 = call-poly <vilib>:"write data element.vi"("value"=w132, "index"=w133, "data table in"=w131) -> ("data table out"=w128:T3)  [unwired: 8 in]
  n94 = call-poly <vilib>:"write data element.vi"("value"=w129, "index"=w130, "data table in"=w128) -> ("data table out"=w125:T3)  [unwired: 8 in]
  n95 = call-poly <vilib>:"write data element.vi"("value"=w126, "index"=w127, "data table in"=w125) -> ("data table out"=w122:T3)  [unwired: 8 in]
  n96 = call-poly <vilib>:"write data element.vi"("value"=w123, "index"=w124, "data table in"=w122) -> ("data table out"=w119:T3)  [unwired: 8 in]
  n97 = call-poly <vilib>:"write data element.vi"("value"=w120, "index"=w121, "data table in"=w119) -> ("data table out"=w116:T3)  [unwired: 8 in]
  n98 = call-poly <vilib>:"write data element.vi"("value"=w117, "index"=w118, "data table in"=w116) -> ("data table out"=w113:T3)  [unwired: 8 in]
  n99 = call-poly <vilib>:"write data element.vi"("value"=w114, "index"=w115, "data table in"=w113) -> ("data table out"=w110:T3)  [unwired: 8 in]
  n100 = call-poly <vilib>:"write data element.vi"("value"=w111, "index"=w112, "data table in"=w110) -> ("data table out"=w107:T3)  [unwired: 8 in]
  n101 = call-poly <vilib>:"write data element.vi"("value"=w108, "index"=w109, "data table in"=w107) -> ("data table out"=w104:T3)  [unwired: 8 in]
  n102 = call-poly <vilib>:"write data element.vi"("value"=w105, "index"=w106, "data table in"=w104) -> ("data table out"=w101:T3)  [unwired: 8 in]
  n103 = call-poly <vilib>:"write data element.vi"("value"=w102, "index"=w103, "data table in"=w101) -> ("data table out"=w98:T3)  [unwired: 8 in]
  n104 = call-poly <vilib>:"write data element.vi"("value"=w99, "index"=w100, "data table in"=w98) -> ("data table out"=w95:T3)  [unwired: 8 in]
  n105 = call-poly <vilib>:"write data element.vi"("value"=w96, "index"=w97, "data table in"=w95) -> ("data table out"=w92:T3)  [unwired: 8 in]
  n106 = call-poly <vilib>:"write data element.vi"("value"=w93, "index"=w94, "data table in"=w92) -> ("data table out"=w89:T3)  [unwired: 8 in]
  n107 = call-poly <vilib>:"write data element.vi"("value"=w90, "index"=w91, "data table in"=w89) -> ("data table out"=w86:T3)  [unwired: 8 in]
  n108 = call-poly <vilib>:"write data element.vi"("value"=w87, "index"=w88, "data table in"=w86) -> ("data table out"=w83:T3)  [unwired: 8 in]
  n109 = call-poly <vilib>:"write data element.vi"("value"=w84, "index"=w85, "data table in"=w83) -> ("data table out"=w80:T3)  [unwired: 8 in]
  n110 = call-poly <vilib>:"write data element.vi"("value"=w81, "index"=w82, "data table in"=w80) -> ("data table out"=w77:T3)  [unwired: 8 in]
  n111 = call-poly <vilib>:"write data element.vi"("value"=w78, "index"=w79, "data table in"=w77) -> ("data table out"=w74:T3)  [unwired: 8 in]
  n112 = call-poly <vilib>:"write data element.vi"("value"=w75, "index"=w76, "data table in"=w74) -> ("data table out"=w71:T3)  [unwired: 8 in]
  n113 = call-poly <vilib>:"write data element.vi"("value"=w72, "index"=w73, "data table in"=w71) -> ("data table out"=w68:T3)  [unwired: 8 in]
  n114 = call-poly <vilib>:"write data element.vi"("value"=w69, "index"=w70, "data table in"=w68) -> ("data table out"=w65:T3)  [unwired: 8 in]
  n115 = call-poly <vilib>:"write data element.vi"("value"=w66, "index"=w67, "data table in"=w65) -> ("data table out"=w62:T3)  [unwired: 8 in]
  n116 = call-poly <vilib>:"write data element.vi"("value"=w63, "index"=w64, "data table in"=w62) -> ("data table out"=w59:T3)  [unwired: 8 in]
  n117 = call-poly <vilib>:"write data element.vi"("value"=w60, "index"=w61, "data table in"=w59) -> ("data table out"=w56:T3)  [unwired: 8 in]
  n118 = call-poly <vilib>:"write data element.vi"("value"=w57, "index"=w58, "data table in"=w56) -> ("data table out"=w53:T3)  [unwired: 8 in]
  n119 = call-poly <vilib>:"write data element.vi"("value"=w54, "index"=w55, "data table in"=w53) -> ("data table out"=w50:T3)  [unwired: 8 in]
  n120 = call-poly <vilib>:"write data element.vi"("value"=w51, "index"=w52, "data table in"=w50) -> ("data table out"=w47:T3)  [unwired: 8 in]
  n121 = call-poly <vilib>:"write data element.vi"("value"=w48, "index"=w49, "data table in"=w47) -> ("data table out"=w44:T3)  [unwired: 8 in]
  n122 = call-poly <vilib>:"write data element.vi"("value"=w45, "index"=w46, "data table in"=w44) -> ("data table out"=w41:T3)  [unwired: 8 in]
  n123 = call-poly <vilib>:"write data element.vi"("value"=w42, "index"=w43, "data table in"=w41) -> ("data table out"=w38:T3)  [unwired: 8 in]
  n124 = call-poly <vilib>:"write data element.vi"("value"=w39, "index"=w40, "data table in"=w38) -> ("data table out"=w35:T3)  [unwired: 8 in]
  n125 = call-poly <vilib>:"write data element.vi"("value"=w36, "index"=w37, "data table in"=w35) -> ("data table out"=w32:T3)  [unwired: 8 in]
  n126 = call-poly <vilib>:"write data element.vi"("value"=w33, "index"=w34, "data table in"=w32) -> ("data table out"=w29:T3)  [unwired: 8 in]
  n127 = call-poly <vilib>:"write data element.vi"("value"=w30, "index"=w31, "data table in"=w29) -> ("data table out"=w26:T3)  [unwired: 8 in]
  n128 = call-poly <vilib>:"write data element.vi"("value"=w27, "index"=w28, "data table in"=w26) -> ("data table out"=w23:T3)  [unwired: 8 in]
  n129 = call-poly <vilib>:"write data element.vi"("value"=w24, "index"=w25, "data table in"=w23) -> ("data table out"=w20:T3)  [unwired: 8 in]
  n130 = call-poly <vilib>:"write data element.vi"("value"=w21, "index"=w22, "data table in"=w20) -> ("data table out"=w17:T3)  [unwired: 8 in]
  n131 = call-poly <vilib>:"write data element.vi"("value"=w18, "index"=w19, "data table in"=w17) -> ("data table out"=w14:T3)  [unwired: 8 in]
  n132 = call-poly <vilib>:"write data element.vi"("value"=w15, "index"=w16, "data table in"=w14) -> ("data table out"=w11:T3)  [unwired: 8 in]
  n133 = call-poly <vilib>:"write data element.vi"("value"=w12, "index"=w13, "data table in"=w11) -> ("data table out"=w8:T3)  [unwired: 8 in]
  n134 = call-poly <vilib>:"write data element.vi"("value"=w9, "index"=w10, "data table in"=w8) -> ("data table out"=w5:T3)  [unwired: 8 in]
  n135 = call-poly <vilib>:"write data element.vi"("value"=w6, "index"=w7, "data table in"=w5) -> ("data table out"=w2:T3)  [unwired: 8 in]
  n136 = call-poly <vilib>:"write data element.vi"("value"=w3, "index"=w4, "data table in"=w2) -> ("data table out"=→"tag bus out":T3)  [unwired: 8 in]
